vi "Replace View into 2D Array.vi"(6 "Directions":T1[](array[typedef])=[enum."NW", enum."N", enum."NE", enum."E", enum."SE", enum."S", enum."S", enum."SW", enum."W"], 8 "View":i32[](array[numeric]), 9 "Column":i32, 10 "Row":i32, 11 "Board Array":i32[][](array[numeric])=[[1, 11, 10, 111, 101], [2, 22, 20, 222, 102], [3, 33, 30, 333, 103], [4, 44, 40, 444, 104], [5, 55, 50, 555, 105]]) -> (3 "Board Array Out":i32[][](array[numeric])=[[1, 11, 10, 111, 101], [2, 22, 20, 222, 102], [3, 33, 30, 333, 103], [4, 44, 40, 444, 104], [5, 55, 50, 555, 105]])   [LabVIEW 2020, in "AntFarm_MB.lvclass"]
uses:
  AntFarm_MB.lvclass
  Type Defs/Direction Enum.ctl
  Type Defs/SB Type Defs.lvlib
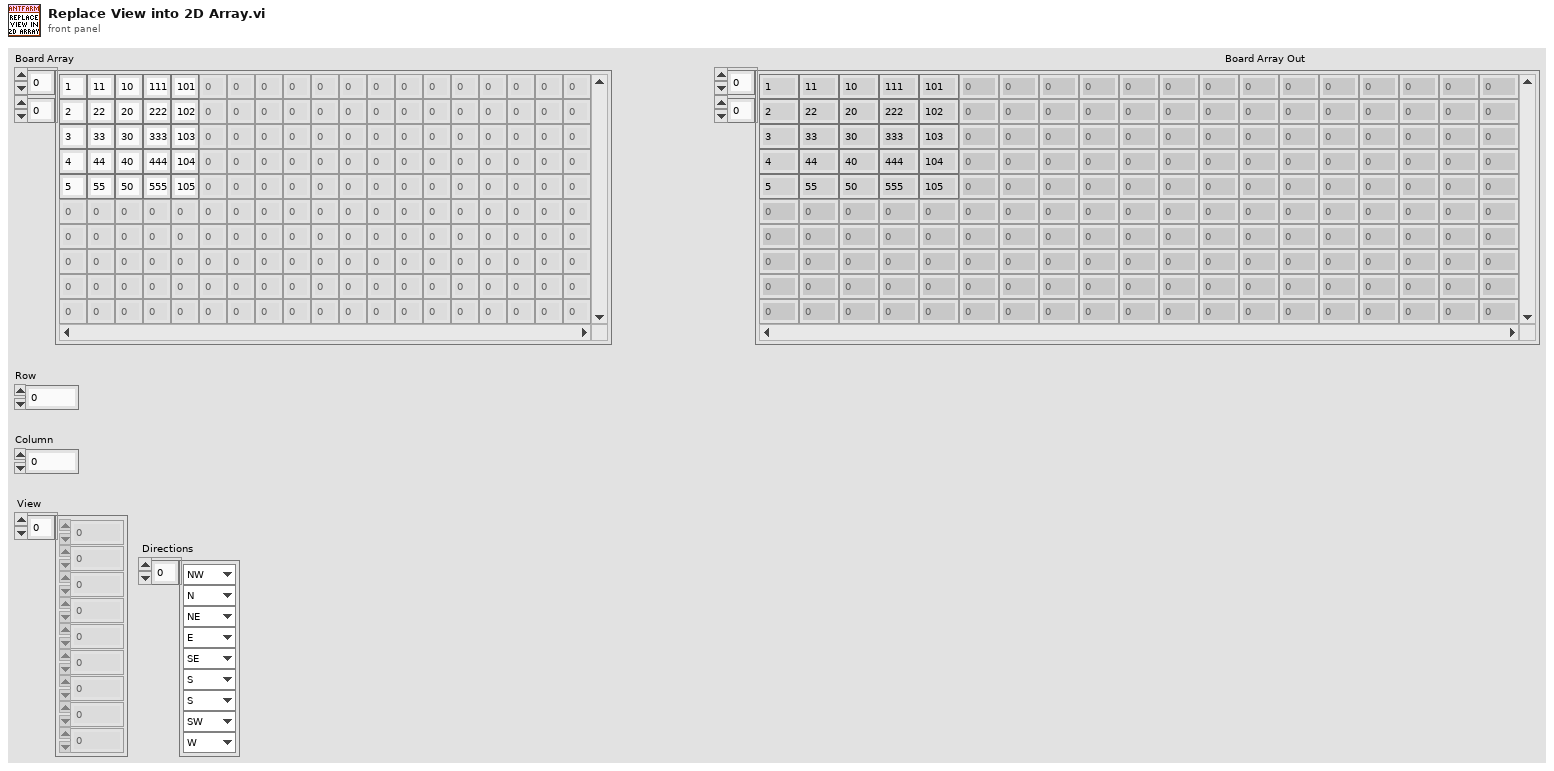
[diagram p1: front panel]
types:
  T1 = typedef "SB Type Defs.lvlib/Direction Enum.ctl" = enum16{"NW", "N", "NE", "E", "SE", "S", "SW", "W"}
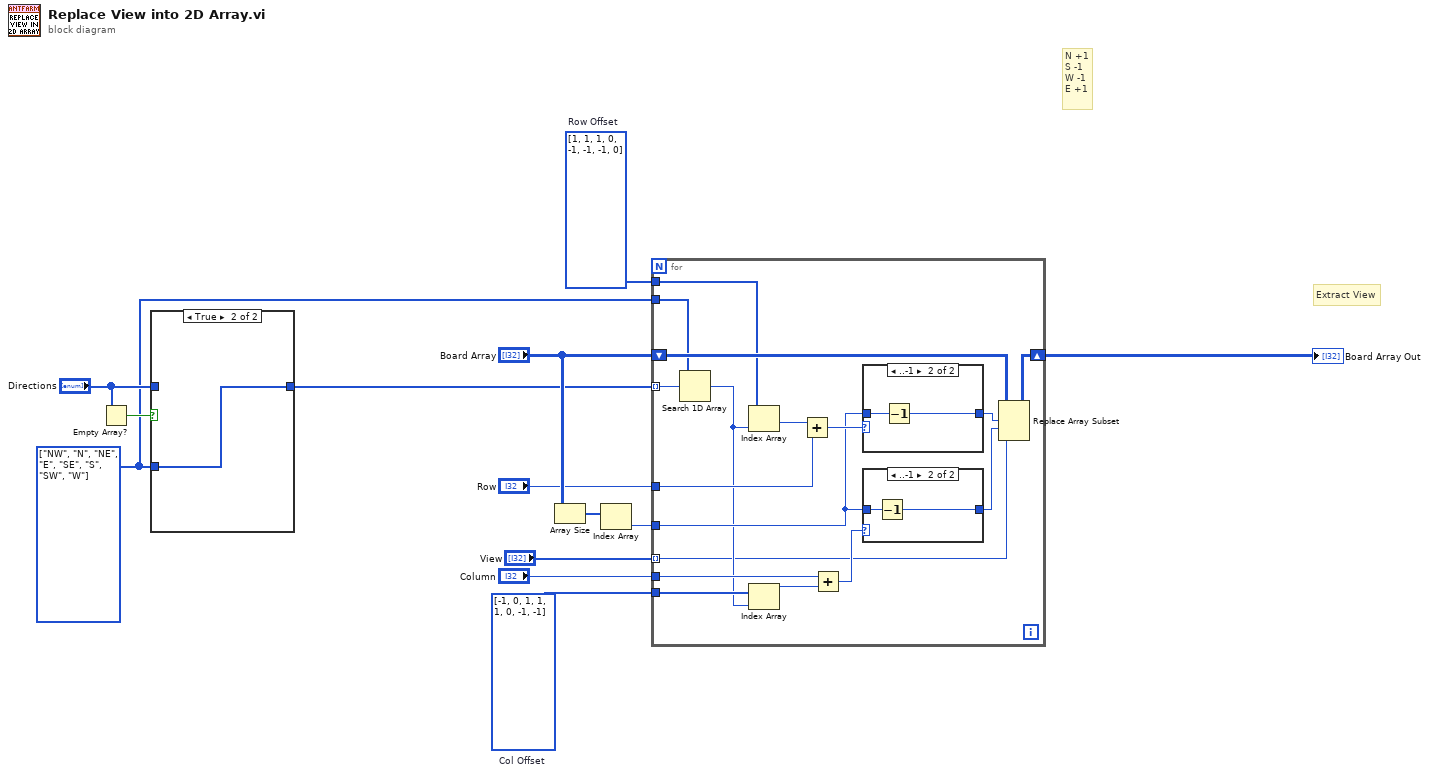
[diagram p0: block diagram]
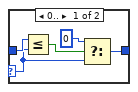
[diagram p3: hidden frame]
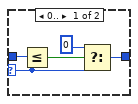
[diagram p4: hidden frame]
diagram:
  w2 = i32[] [-1, 0, 1, 1, 1, 0, -1, -1]  # Col Offset
  w1 = i32[] [1, 1, 1, 0, -1, -1, -1, 0]  # Row Offset
  w3 = T1[] [enum."NW", enum."N", enum."NE", enum."E", enum."SE", enum."S", enum."SW", enum."W"] items=["NW", "N", "NE", "E", "SE", "S", "SW", "W"] ("Directions Out")
  # "N +1\nS -1\nW -1\nE +1"
  # "Extract View"
  n1 = Empty Array?(array="Directions") -> (empty?=w7:bool)
  n2 = case shown="True" w7 {
    tunnel: "Directions" -> [w14 _]
    tunnel: [w14 w15] -> w5
    tunnel: w3 -> [_ w15]
    frame False {
    }
    frame True {
    }
  }
  n3 = Array Size(array="Board Array") -> (size(s)=w10:i32[])
  n4 = Index Array(array=w10) -> (element=w9:i32)  [unwired: 1 in]
  n5 = for {
    tunnel: w9 -> [w28]
    tunnel: "Row" -> [w32]
    tunnel: "Column" -> [w30]
    shift-right: [w25] -> w8
    shift-left: "Board Array" -> [w27]
    tunnel: w5 -> [w22] mode=indexing
    tunnel: "View" -> [w16] mode=indexing
    tunnel: w3 -> [w23]
    tunnel: w2 -> [w21]
    tunnel: w1 -> [w19]
    n6 = Search 1D Array(1D array=w23, element=w22) -> (index of element=w18:i32)  [unwired: 1 in]
    n7 = Index Array(array=w19, index=w18) -> (element=w17:i32)
    n8 = Index Array(array=w21, index=w18) -> (element=w20:i32)
    n9 = Add(x=w17, y=w32) -> (x+y=w31:i32)
    n10 = Add(x=w30, y=w20) -> (x+y=w29:i32)
    n11 = case shown="..-1" w31 {
      selector: w31 -> [w42 _]
      tunnel: w28 -> [w41 w46]
      tunnel: [w40 w45] -> w26
      frame 0.. {
        n12 = Less Or Equal?(x=w41, y=w42) -> (x <= y?=w43:bool)
        n13 = Select(t=0, s=w43, f=w42) -> (s? t:f=w40:i32)
      }
      frame ..-1 {
        n14 = Decrement(x=w46) -> (x-1=w45:i32)
      }
    }
    n15 = case shown="..-1" w29 {
      selector: w29 -> [w35 _]
      tunnel: w28 -> [w37 w39]
      tunnel: [w34 w38] -> w24
      frame 0.. {
        n16 = Less Or Equal?(x=w37, y=w35) -> (x <= y?=w36:bool)
        n17 = Select(t=0, s=w36, f=w35) -> (s? t:f=w34:i32)
      }
      frame ..-1 {
        n18 = Decrement(x=w39) -> (x-1=w38:i32)
      }
    }
    n19 = Replace Array Subset(array=w27, new element=w16, index (row)=w26, index (col)=w24) -> (w25:i32[][])
  }
  "Board Array Out" <- w8
